vi "List Keys.vi"(7 "Section":string, 8 "error in (no error)":errorcluster, 11 "Ini Path in":path) -> (0 "error out":errorcluster, 1 "Section Found?":bool, 2 "Keys":string[](array[string]), 3 "Ini Path out":path)   [LabVIEW 2018, in "Config.lvlib"]
uses:
  Config.lvlib
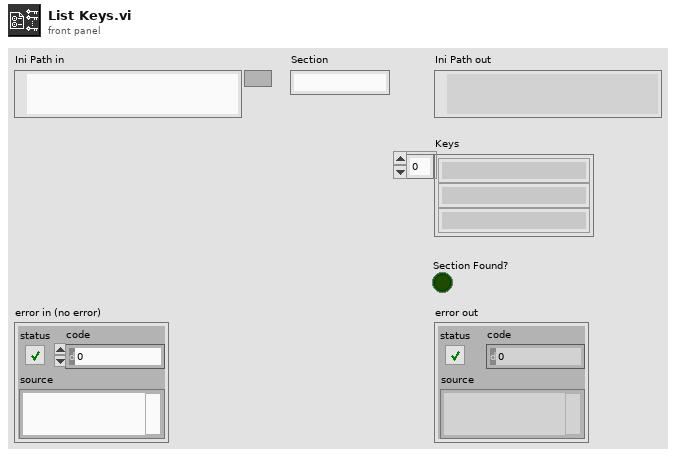
[diagram p1: front panel]
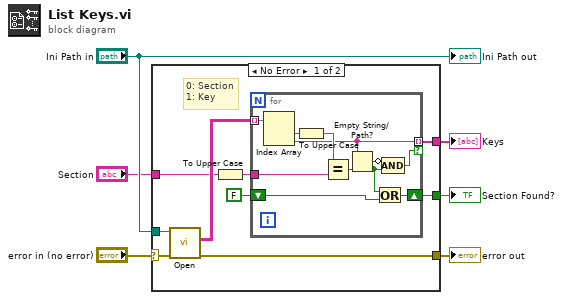
[diagram p0: block diagram]
diagram:
  n1 = case shown="No Error" "error in (no error)" {
    selector: "error in (no error)" -> [w15 w26]
    tunnel: [w14 w26] -> w5
    tunnel: "Ini Path in" -> [w13 _]
    tunnel: "Section" -> [w9 _]
    tunnel: [w8 _] -> w2
    tunnel: [w7 _] -> w1
    frame No Error {
      # "0: Section\n1: Key"
      n2 = call "Open.vi"("error in (no error)"=w15, "Ini Path in"=w13) -> ("error out"=w14:errorcluster, "skvc out"=w10:string[][])  [unwired: 6 in, 2 out]
      n3 = To Upper Case(1:w9) -> (0:w12:string)
      n4 = for {
        tunnel: w10 -> [w25] mode=indexing
        tunnel: [w21] -> w8 mode=indexing if=w19
        tunnel: w12 -> [w22]
        shift-right: [w17] -> w7
        shift-left: FALSE -> [w16]
        n5 = Index Array(array=w25) -> (element #1=w24:string, element #2=w21:string)  [unwired: 2 in]
        n6 = To Upper Case(1:w24) -> (0:w23:string)
        n7 = Equal?(x=w23, y=w22) -> (x = y?=w18:bool)
        n8 = Empty String/Path?(string/path=w21) -> (empty?=w20:bool)
        n9 = Or(x=w18, y=w16) -> (x .or. y?=w17:bool)
        n10 = Compound Arithmetic op=AND(invert w20, w18) -> (w19:bool)
      }
    }
    frame Error {
    }
  }
  "error out" <- w5
  "Keys" <- w2
  "Section Found?" <- w1
  "Ini Path out" <- "Ini Path in"
